vi "Get Data from SLSC.vi"(8 "error in (no error)":errorcluster, 11 "SLSC Switch in":refnum<class "SLSC Switch.lvclass">) -> (0 "error out":errorcluster, 3 "SLSC Switch out":refnum<class "SLSC Switch.lvclass">)   [LabVIEW 2015, in "SLSC Switch.lvclass"]
uses:
  SLSC Switch.lvclass
  SLSC Switch.lvclass/SLSC Switch.ctl
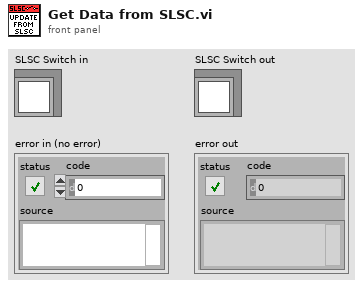
[diagram p1: front panel]
types:
  T1 = typedef "SLSC Switch.lvclass/Topology.ctl" = cluster{"Topology Name":string, "Topology File Path":path, "Channels":string[]}
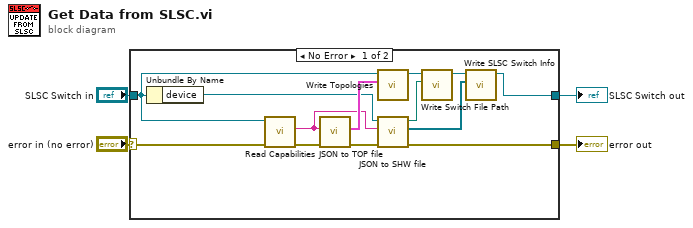
[diagram p0: block diagram]
diagram:
  n1 = case shown="No Error" "error in (no error)" {
    selector: "error in (no error)" -> [w10 w19]
    tunnel: [w14 w19] -> w3
    tunnel: "SLSC Switch in" -> [w8 w18]
    tunnel: [w5 w18] -> w1
    frame No Error {
      n2 = Unbundle By Name(w8) -> ("device"=w7:refnum<k21>)
      n3 = call "Read Capabilities.vi"("error in (no error)"=w10, "SLSC Switch in"=w8) -> ("error out"=w9:errorcluster, "capabilities"=w6:string)  [unwired: 8 in]
      n4 = call "JSON to TOP file.vi"("error in (no error)"=w9, "Capabilities JSON In"=w6) -> ("error out"=w15:errorcluster, "Topologies out"=w16:T1[])  [unwired: 8 in]
      n5 = call "Write Topologies.vi"("Topologies"=w16, "SLSC Switch in"=w8) -> ("SLSC Switch out"=w17:refnum<class "SLSC Switch.lvclass">)  [unwired: 9 in]
      n6 = call "JSON to SHW file.vi"("error in (no error)"=w15, "Capabilities JSON In"=w6, "device"=w7) -> ("error out"=w14:errorcluster, "SLSC Switch Info"=w11:refnum<class "RelayInterface.lvclass">[], "SHW Path Out"=w12:path)  [unwired: 6 in]
      n7 = call "Write Switch File Path.vi"("Switch File Path"=w12, "SLSC Switch in"=w17) -> ("SLSC Switch out"=w13:refnum<class "SLSC Switch.lvclass">)  [unwired: 9 in]
      n8 = call "Write SLSC Switch Info.vi"("SLSC Switch Info"=w11, "SLSC Switch in"=w13) -> ("SLSC Switch out"=w5:refnum<class "SLSC Switch.lvclass">)  [unwired: 9 in]
    }
    frame Error {
    }
  }
  "error out" <- w3
  "SLSC Switch out" <- w1
